vi "Convert Write ERD List to Message (Rev 2 API).vi"(0 "GEA Inputs":T3 {"Destination" format="%.0x"; "Source" format="%.0x"}, 7 "ERD Read Data In":T1 {"ERD Number" format="%.0x"}, 11 "Error In":errorcluster) -> (4 "GEA Message":T4 {"Command" format="%02x"; "Destination" format="%02x"; "Source" format="%02x"}, 6 "Request ID":string, 15 "Error Out":errorcluster)   [LabVIEW 2023, in "GEA2_Toolkit.lvlib"]
doc: "This vi uses the Source / Destination from the GEA input and the ERD Write list to format a single GEA2 message to read the list of ERDs."
uses:
  library/GEA2_Toolkit.lvlib
  type defs/Data In.ctl
  type defs/Source_Destination.ctl
  type defs/ERD Write Data In.ctl
  type defs/Data Type.ctl
  <vilib>/regexp/Match Regular Expression.xnode
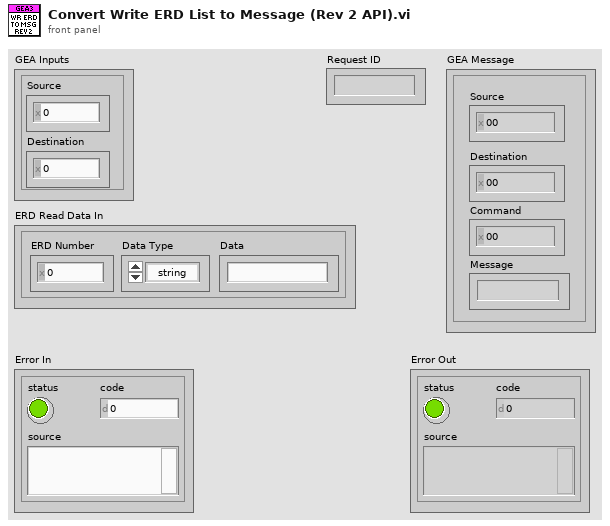
[diagram p1: front panel]
types:
  T1 = typedef "GEA2_Toolkit.lvlib/ERD Write Data In.ctl" = cluster{"ERD Number":u16, "Data Type":T2, "Data":string}
  T2 = typedef "GEA2_Toolkit.lvlib/Data Type.ctl" = enum16{"string", "boolean", "uint8_t", "uint16_t", "uint32_t", "uint64_t", "int8_t", "int16_t", "int32_t", "int64_t"}
  T3 = typedef "GEA2_Toolkit.lvlib/Source_Destination.ctl" = cluster{"Source":u8, "Destination":u8}
  T4 = typedef "GEA2_Toolkit.lvlib/Data In.ctl" = cluster{"Source":u8, "Destination":u8, "Command":u8, "Message":string}
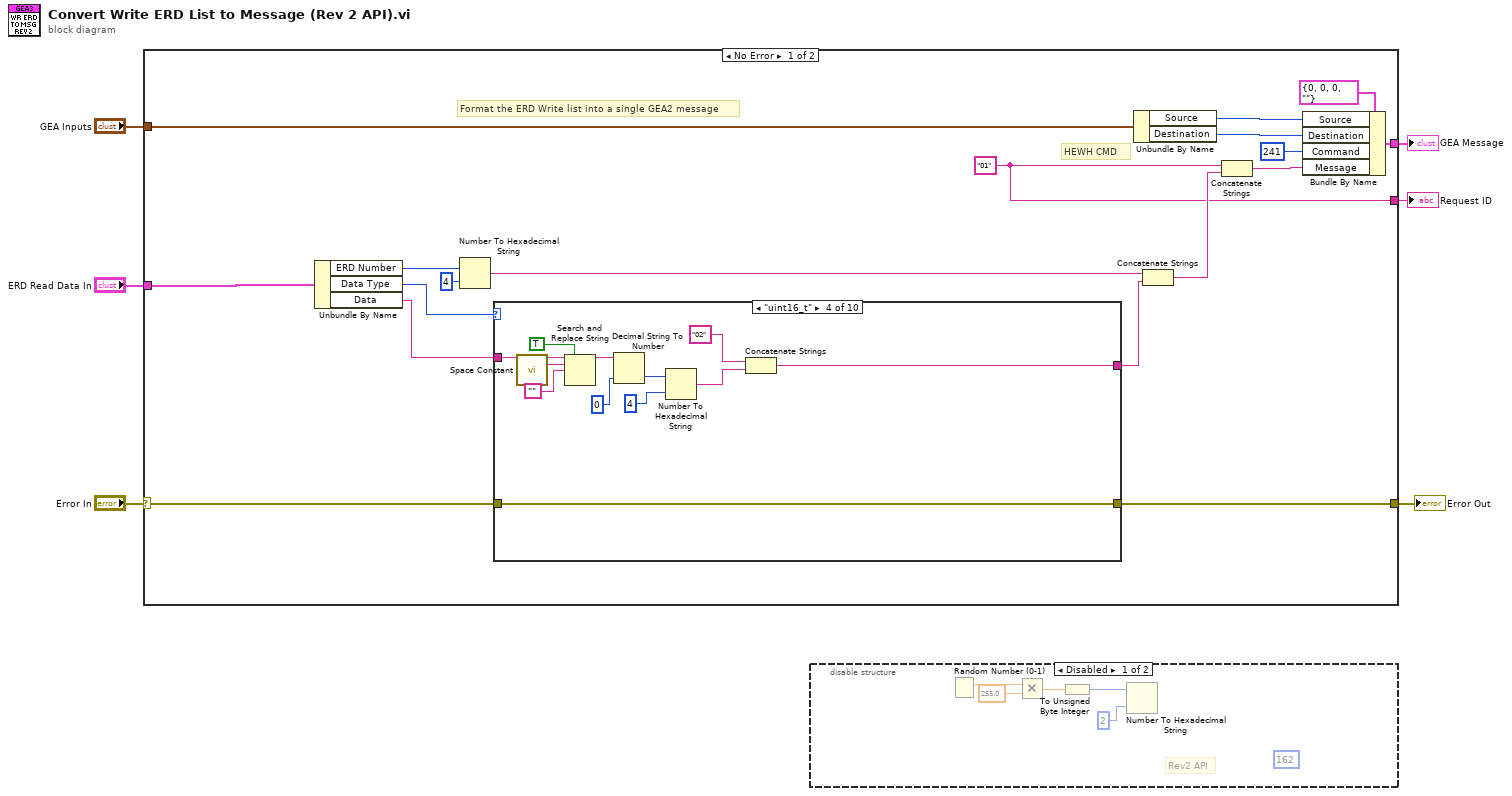
[diagram p0: block diagram]
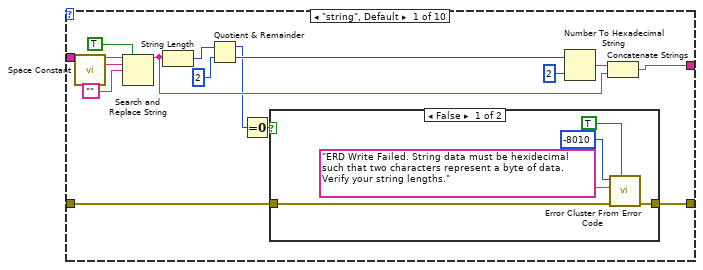
[diagram p3: hidden frame]
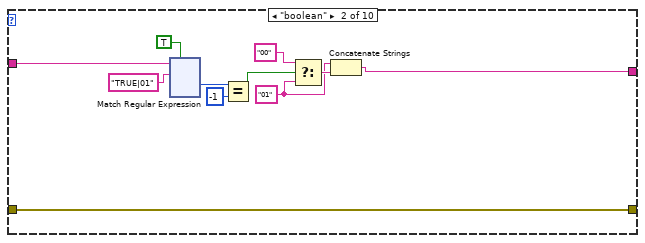
[diagram p5: hidden frame]
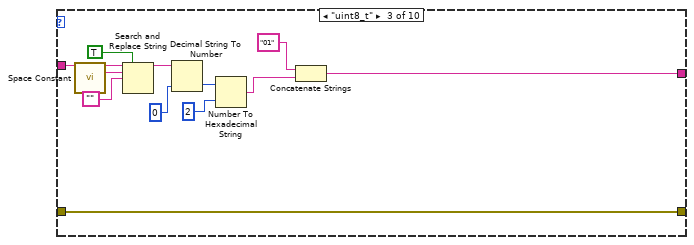
[diagram p6: hidden frame]
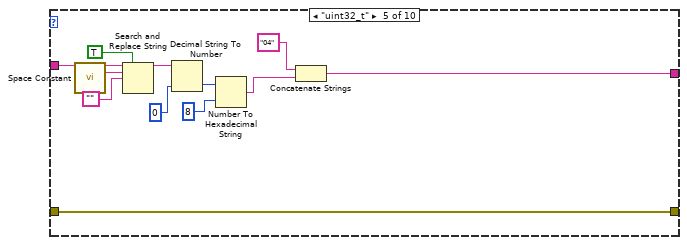
[diagram p7: hidden frame]
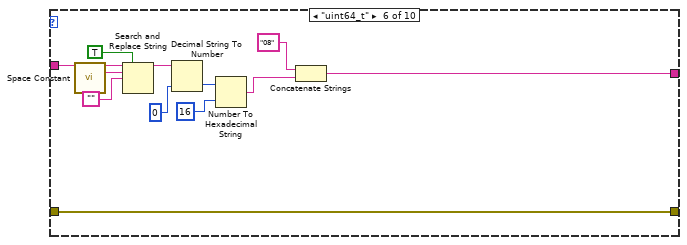
[diagram p8: hidden frame]
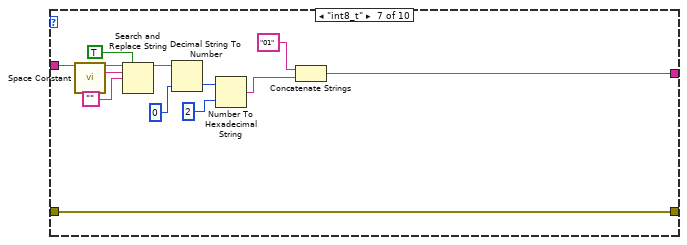
[diagram p9: hidden frame]
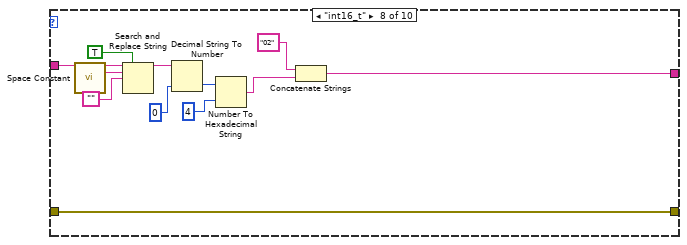
[diagram p10: hidden frame]
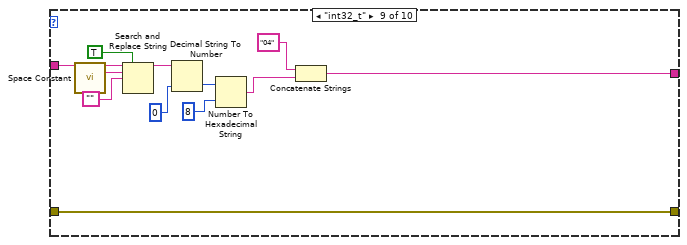
[diagram p11: hidden frame]
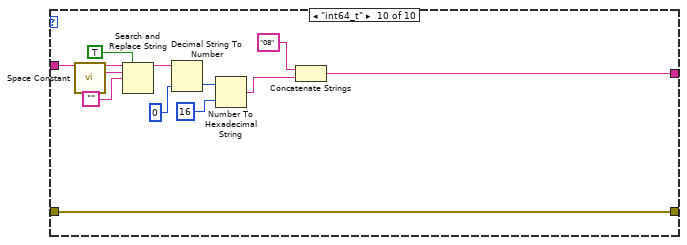
[diagram p12: hidden frame]
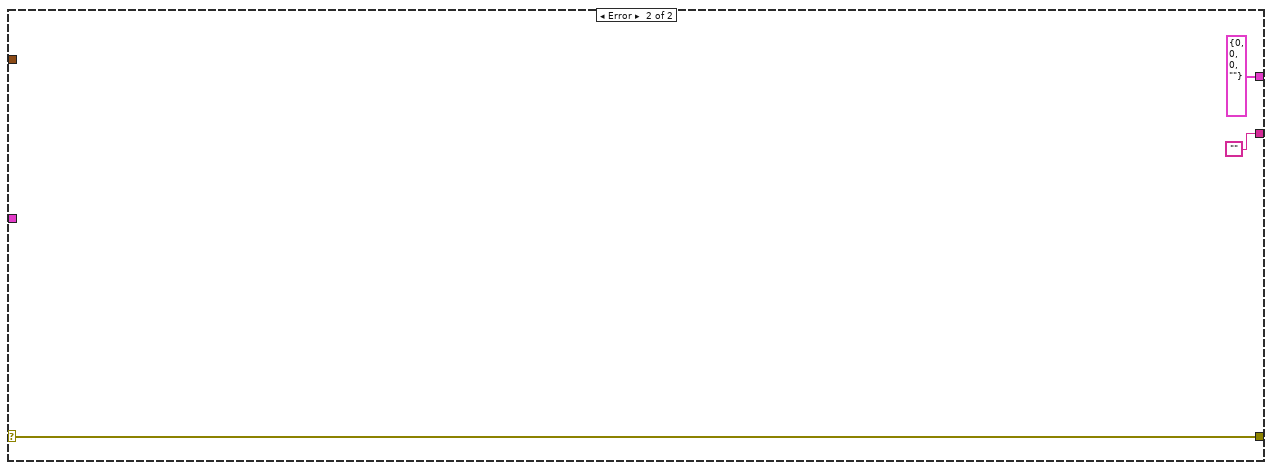
[diagram p13: hidden frame]
diagram:
  n1 = case shown="No Error" "Error In" {
    selector: "Error In" -> [w16 w272]
    tunnel: "GEA Inputs" -> [w22 _]
    tunnel: [w17 T4 {"Source"=0, "Destination"=0, "Command"=0, "Message"=""} ("GEA Message")] -> w5
    tunnel: [w15 w272] -> w3
    tunnel: [w7 ""] -> w2
    tunnel: "ERD Read Data In" -> [w8 _]
    frame No Error {
      w7 = "01"
      # "HEWH CMD"
      # "Format the ERD Write list into a single GEA2 message"
      n2 = Unbundle By Name(w8) -> ("ERD Number"=w14:u16, "Data Type"=w11:T2, "Data"=w10:string)
      n3 = Number To Hexadecimal String(1:i16 4 ("width (-)"), 2:w14) -> (0:w12:string)
      n4 = case shown="\"uint16_t\"" w11 {
        tunnel: w10 -> [w39 w55 w182 w187 w200 w212 w224 w236 w248 w260]
        tunnel: [w34 w48 w181 w188 w199 w211 w223 w235 w247 w259] -> w9
        tunnel: w16 -> [w28 w46 w174 w186 w198 w210 w222 w234 w246 w258]
        tunnel: [w25 w46 w174 w186 w198 w210 w222 w234 w246 w258] -> w15
        frame "string", Default {
          n5 = call <vilib>:"Space Constant.vi"() -> ("String"=w37:string)
          n6 = Search and Replace String(replace all?=TRUE ("replace all? (F)"), input string=w39, search string=w37, replace string="") -> (result string=w33:string)  [unwired: 4 in, 3 out]
          n7 = String Length(string=w33) -> (length=w31:i32)
          n8 = Quotient & Remainder(x=w31, y=2) -> (x-y*floor(x/y)=w27:i32, floor(x/y)=w30:i32)
          n9 = Equal To 0?(x=w27) -> (x = 0?=w26:bool)
          n10 = case shown="False" w26 {
            tunnel: w28 -> [w44 w45]
            tunnel: [w40 w45] -> w25
            frame False {
              n11 = call <vilib>:"Error Cluster From Error Code.vi"("show call chain? (False)"=TRUE, "error in (no error)"=w44, "error message (\"\")"="ERD Write Failed. String data must be hexidecimal such that two characters represent a byte of data. Verify your string lengths." ("error message (\"\")"), "error code (0)"=-8010) -> ("error out"=w40:errorcluster)  [unwired: 5 in]
            }
            frame True {
            }
          }
          n12 = Number To Hexadecimal String(1:i16 2 ("width (-)"), 2:w30) -> (0:w35:string)
          n13 = Concatenate Strings(w35, w33) -> (w34:string)
        }
        frame "boolean" {
          w47 = "01"
          n14 = xnode "Match Regular Expression"("input string"=w55, "regular expression"="TRUE|01", "ignore case? (F)"=TRUE) -> ("offset past match"=w53:i32)  [unwired: 3 in, 4 out]
          n15 = Equal?(x=w53, y=-1) -> (x = y?=w50:bool)
          n16 = Select(t="00", s=w50, f=w47) -> (s? t:f=w49:string)
          n17 = Concatenate Strings(w47, w49) -> (w48:string)
        }
        frame "uint8_t" {
          n18 = call <vilib>:"Space Constant.vi"() -> ("String"=w184:string)
          n19 = Search and Replace String(replace all?=TRUE ("replace all? (F)"), input string=w182, search string=w184, replace string="") -> (result string=w179:string)  [unwired: 4 in, 3 out]
          n20 = Decimal String To Number(string=w179, default (0L)=u8 0) -> (number=w176:u8)  [unwired: 1 in, 1 out]
          n21 = Number To Hexadecimal String(1:i16 2 ("width (-)"), 2:w176) -> (0:w175:string)
          n22 = Concatenate Strings("01", w175) -> (w181:string)
        }
        frame "uint16_t" {
          n23 = call <vilib>:"Space Constant.vi"() -> ("String"=w196:string)
          n24 = Search and Replace String(replace all?=TRUE ("replace all? (F)"), input string=w187, search string=w196, replace string="") -> (result string=w193:string)  [unwired: 4 in, 3 out]
          n25 = Decimal String To Number(string=w193, default (0L)=u16 0) -> (number=w190:u16)  [unwired: 1 in, 1 out]
          n26 = Number To Hexadecimal String(1:i16 4 ("width (-)"), 2:w190) -> (0:w189:string)
          n27 = Concatenate Strings("02", w189) -> (w188:string)
        }
        frame "uint32_t" {
          n28 = call <vilib>:"Space Constant.vi"() -> ("String"=w208:string)
          n29 = Search and Replace String(replace all?=TRUE ("replace all? (F)"), input string=w200, search string=w208, replace string="") -> (result string=w205:string)  [unwired: 4 in, 3 out]
          n30 = Decimal String To Number(string=w205, default (0L)=u32 0) -> (number=w202:u32)  [unwired: 1 in, 1 out]
          n31 = Number To Hexadecimal String(1:i16 8 ("width (-)"), 2:w202) -> (0:w201:string)
          n32 = Concatenate Strings("04", w201) -> (w199:string)
        }
        frame "uint64_t" {
          n33 = call <vilib>:"Space Constant.vi"() -> ("String"=w220:string)
          n34 = Search and Replace String(replace all?=TRUE ("replace all? (F)"), input string=w212, search string=w220, replace string="") -> (result string=w217:string)  [unwired: 4 in, 3 out]
          n35 = Decimal String To Number(string=w217, default (0L)=u64 0) -> (number=w214:u64)  [unwired: 1 in, 1 out]
          n36 = Number To Hexadecimal String(1:i16 16 ("width (-)"), 2:w214) -> (0:w213:string)
          n37 = Concatenate Strings("08", w213) -> (w211:string)
        }
        frame "int8_t" {
          n38 = call <vilib>:"Space Constant.vi"() -> ("String"=w232:string)
          n39 = Search and Replace String(replace all?=TRUE ("replace all? (F)"), input string=w224, search string=w232, replace string="") -> (result string=w229:string)  [unwired: 4 in, 3 out]
          n40 = Decimal String To Number(string=w229, default (0L)=i8 0) -> (number=w226:i8)  [unwired: 1 in, 1 out]
          n41 = Number To Hexadecimal String(1:i16 2 ("width (-)"), 2:w226) -> (0:w225:string)
          n42 = Concatenate Strings("01", w225) -> (w223:string)
        }
        frame "int16_t" {
          n43 = call <vilib>:"Space Constant.vi"() -> ("String"=w244:string)
          n44 = Search and Replace String(replace all?=TRUE ("replace all? (F)"), input string=w236, search string=w244, replace string="") -> (result string=w241:string)  [unwired: 4 in, 3 out]
          n45 = Decimal String To Number(string=w241, default (0L)=i16 0) -> (number=w238:i16)  [unwired: 1 in, 1 out]
          n46 = Number To Hexadecimal String(1:i16 4 ("width (-)"), 2:w238) -> (0:w237:string)
          n47 = Concatenate Strings("02", w237) -> (w235:string)
        }
        frame "int32_t" {
          n48 = call <vilib>:"Space Constant.vi"() -> ("String"=w256:string)
          n49 = Search and Replace String(replace all?=TRUE ("replace all? (F)"), input string=w248, search string=w256, replace string="") -> (result string=w253:string)  [unwired: 4 in, 3 out]
          n50 = Decimal String To Number(string=w253, default (0L)=0) -> (number=w250:i32)  [unwired: 1 in, 1 out]
          n51 = Number To Hexadecimal String(1:i16 8 ("width (-)"), 2:w250) -> (0:w249:string)
          n52 = Concatenate Strings("04", w249) -> (w247:string)
        }
        frame "int64_t" {
          n53 = call <vilib>:"Space Constant.vi"() -> ("String"=w268:string)
          n54 = Search and Replace String(replace all?=TRUE ("replace all? (F)"), input string=w260, search string=w268, replace string="") -> (result string=w265:string)  [unwired: 4 in, 3 out]
          n55 = Decimal String To Number(string=w265, default (0L)=i64 0) -> (number=w262:i64)  [unwired: 1 in, 1 out]
          n56 = Number To Hexadecimal String(1:i16 16 ("width (-)"), 2:w262) -> (0:w261:string)
          n57 = Concatenate Strings("08", w261) -> (w259:string)
        }
      }
      n58 = Unbundle By Name(w22) -> ("Source"=w21:u8, "Destination"=w20:u8)
      n59 = Concatenate Strings(w12, w9) -> (w24:string)
      n60 = Concatenate Strings(w7, w24) -> (w18:string)
      n61 = Bundle By Name(cluster=T4 {"Source"=0, "Destination"=0, "Command"=0, "Message"=""} ("GEA Message"), "Source"=w21, "Destination"=w20, "Command"=u8 241, "Message"=w18) -> (w17:T4)
    }
    frame Error {
    }
  }
  "GEA Message" <- w5
  "Error Out" <- w3
  "Request ID" <- w2
  n62 = disable-structure shown="Disabled" {
    frame Disabled {
      (unwired) u8 162 ("Command")
      # "Rev2 API"
      n63 = Random Number (0-1)() -> (number: 0 to 1=w273:dbl)
      n64 = Multiply(x=w273, y=255.0) -> (x*y=w275:dbl)
      n65 = To Unsigned Byte Integer(number=w275) -> (unsigned 8bit integer=w276:u8)
      n66 = Number To Hexadecimal String(1:i16 2 ("width (-)"), 2:w276) -> ()  [unwired: 1 out]
    }
    frame Enabled {
    }
  }
